vi "Get All RFmx Sessions and Test Info with Tester Type.vi"(0 "TSM Context In":T1, 5 "Tester Type":string="RFPM", 11 "error in":errorcluster) -> (4 "TSM Context Out":T1, 6 "RFmx Sessions":refnum<k21>[](array[refnum]), 8 "Resource Descriptors":string[](array[string]), 10 "Instrument Models":string[](array[string]), 15 "error out":errorcluster)   [LabVIEW 2023, in "RFCalAndFixtureCharact.Common.lvlib"]
uses:
  RFCalAndFixtureCharact.Common.lvlib
  <vilib>/NI_TestStand_SemiconductorModule/NI_TestStand_Semiconductor_Module.lvlibp/PinMap/General/SemiconductorModuleContext.ctl
  Global Data Id Prefix.vi
  <vilib>/NI_TestStand_SemiconductorModule/NI_TestStand_Semiconductor_Module.lvlibp/PinMap/Site and Global Data/GlobalDataExists.vi
  <vilib>/NI_TestStand_SemiconductorModule/NI_TestStand_Semiconductor_Module.lvlibp/PinMap/Site and Global Data/GetGlobalData.vi
  <vilib>/Utility/error.llb/Error Cluster From Error Code.vi
  <vilib>/ErrorRing/Error Ring.xnode
  <vilib>/NI_TestStand_SemiconductorModule/NI_TestStand_Semiconductor_Module.lvlibp
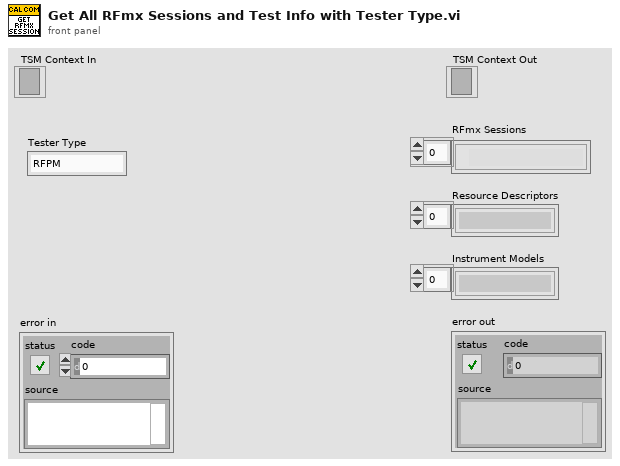
[diagram p1: front panel]
types:
  T1 = typedef "NI_TestStand_Semiconductor_Module.lvlibp/SemiconductorModuleContext.ctl" = refnum<k7>
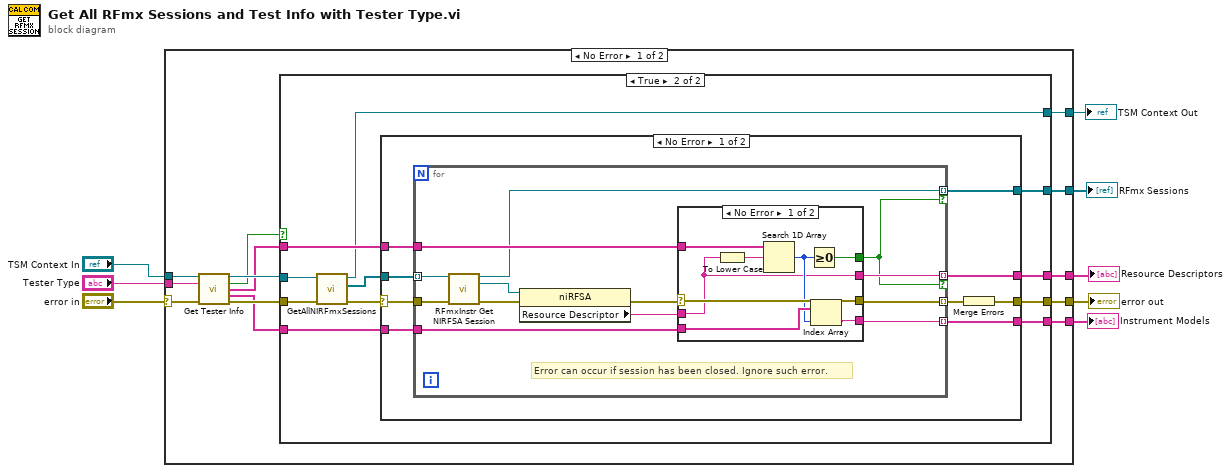
[diagram p0: block diagram]
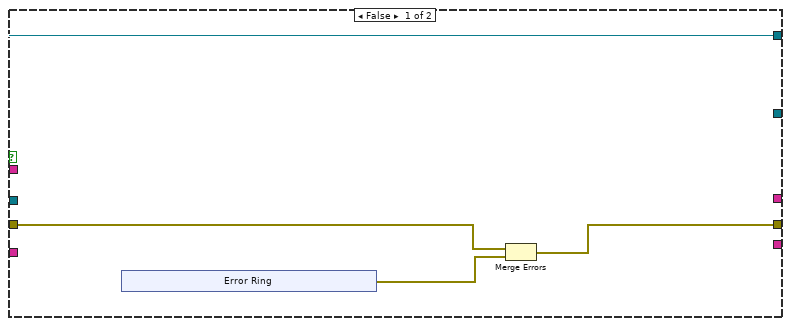
[diagram p2: hidden frame]
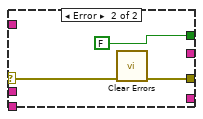
[diagram p3: hidden frame]
diagram:
  n1 = case shown="No Error" "error in" {
    selector: "error in" -> [w14 w76]
    tunnel: "TSM Context In" -> [w21 w77]
    tunnel: [w20 w76] -> w7
    tunnel: [w19 _] -> w6
    tunnel: "Tester Type" -> [w18 _]
    tunnel: [w17 w77] -> w4
    tunnel: [w13 _] -> w2
    tunnel: [w12 _] -> w1
    frame No Error {
      n2 = call "Get Tester Info.vi"("TSM Context In"=w21, "Tester Type"=w18, "error in"=w14) -> ("TSM Context Out"=w15:T1, "Resource Descriptors Exist?"=w11:bool, "Resource Descriptors"=w10:string[], "Instrument Models"=w9:string[], "error out"=w16:errorcluster)  [unwired: 8 in]
      n3 = case shown="True" w11 {
        tunnel: w10 -> [_ w41]
        tunnel: w16 -> [w23 w34]
        tunnel: [w24 w40] -> w20
        tunnel: [_ w39] -> w19
        tunnel: w15 -> [w22 w33]
        tunnel: [w22 w36] -> w17
        tunnel: w9 -> [_ w35]
        tunnel: [_ w32] -> w13
        tunnel: [_ w31] -> w12
        frame False {
          n4 = xnode "Error Ring"() -> ("error out"=w25:errorcluster)
          n5 = Merge Errors(w23, w25) -> (w24:errorcluster)
        }
        frame True {
          n6 = call <vilib>:"GetAllNIRFmxSessions.vi"("error in (no error)"=w34, "Semiconductor Module Context"=w33) -> ("error out"=w37:errorcluster, "Instrument Sessions"=w38:refnum<k21>[], "Semiconductor Module Context Out"=w36:T1)  [unwired: 7 in]
          n7 = case shown="No Error" w37 {
            selector: w37 -> [w48 w75]
            tunnel: w38 -> [w50 _]
            tunnel: w41 -> [w49 _]
            tunnel: [w46 w75] -> w40
            tunnel: [w45 _] -> w39
            tunnel: w35 -> [w44 _]
            tunnel: [w43 _] -> w32
            tunnel: [w42 _] -> w31
            frame No Error {
              n8 = for {
                tunnel: w48 -> [w63]
                tunnel: w50 -> [w62] mode=indexing
                tunnel: w49 -> [w57]
                tunnel: [w56] -> w45 mode=indexing if=w51
                tunnel: [w55] -> w47 mode=indexing
                tunnel: w44 -> [w54]
                tunnel: [w53] -> w43 mode=indexing
                tunnel: [w52] -> w42 mode=indexing if=w51
                # "Error can occur if session has been closed. Ignore such error."
                n9 = call <vilib>:"RFmxInstr Get NIRFSA Session.vi"("Instrument Handle In"=w62, "error in (no error)"=w63) -> ("Instrument Handle Out"=w56:refnum<k21>, "NI RFSA Session"=w60:refnum<k15>, "error out"=w61:errorcluster)  [unwired: 11 in]
                n10 = property class="niRFSA"(reference=w60, error in=w61) -> (error out=w59:errorcluster, "Resource Descriptor"=w58:string)  [unwired: 1 out]
                n11 = case shown="No Error" w59 {
                  selector: w59 -> [w68 w73]
                  tunnel: w58 -> [w64 _]
                  tunnel: w57 -> [w71 _]
                  tunnel: [w70 FALSE] -> w51
                  tunnel: [w68 w72] -> w55
                  tunnel: w54 -> [w67 _]
                  tunnel: [w65 _] -> w53
                  tunnel: [w64 _] -> w52
                  frame No Error {
                    n12 = To Lower Case(string=w64) -> (all lower case string=w69:string)
                    n13 = Search 1D Array(1D array=w71, element=w69) -> (index of element=w66:i32)  [unwired: 1 in]
                    n14 = Greater Or Equal To 0?(x=w66) -> (x >= 0?=w70:bool)
                    n15 = Index Array(array=w67, index=w66) -> (element=w65:string)
                  }
                  frame Error {
                    n16 = call <vilib>:"Clear Errors.vi"("error in (no error)"=w73) -> ("error out"=w72:errorcluster)  [unwired: 5 in, 1 out]
                  }
                }
              }
              n17 = Merge Errors(w47) -> (w46:errorcluster)
            }
            frame Error {
            }
          }
        }
      }
    }
    frame Error {
    }
  }
  "TSM Context Out" <- w4
  "error out" <- w7
  "RFmx Sessions" <- w6
  "Instrument Models" <- w2
  "Resource Descriptors" <- w1
